vi "Switch Columns between Test tables.vi"(7 "New Table":string, 8 "error in (no error)":errorcluster, 9 "Old Column":string, 10 "Old Table":string, 11 "LV-Data.PGSQL in":refnum<class "LV-Data.PGSQL.lvclass">) -> (0 "error out":errorcluster, 2 "Result":string[][](array[string]), 3 "LV-Data.PGSQL out":refnum<class "LV-Data.PGSQL.lvclass">)   [LabVIEW 2016]
uses:
  LV-Data/src/LV-Data.PG/LV-Data.PGSQL.lvclass
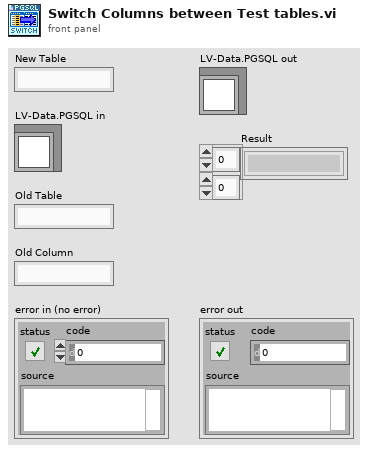
[diagram p1: front panel]
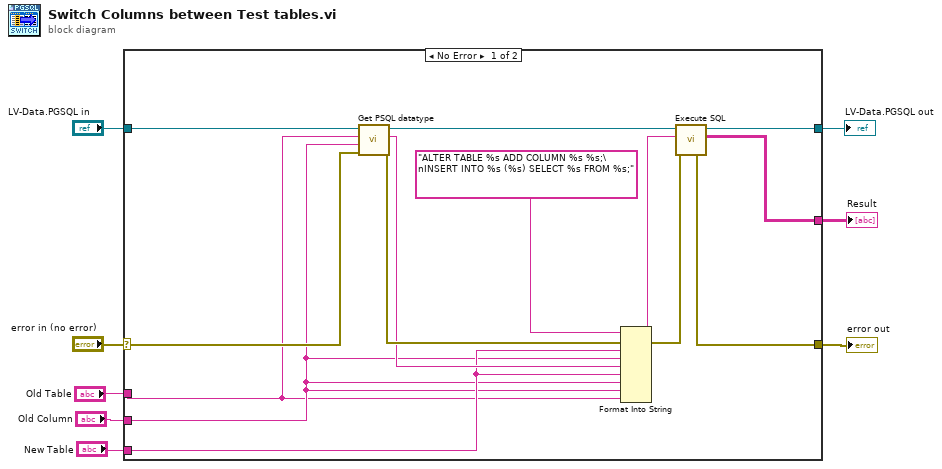
[diagram p0: block diagram]
diagram:
  n1 = case shown="No Error" "error in (no error)" {
    selector: "error in (no error)" -> [w16 w23]
    tunnel: "New Table" -> [w11 _]
    tunnel: "Old Column" -> [w10 _]
    tunnel: "LV-Data.PGSQL in" -> [w15 w24]
    tunnel: [w21 w23] -> w7
    tunnel: [w22 w24] -> w3
    tunnel: "Old Table" -> [w9 _]
    tunnel: [w19 _] -> w8
    frame No Error {
      n2 = call "Get PSQL datatype.vi"("error in (no error)"=w16, "Column"=w10, "Table"=w9, "LV-Data.PGSQL in"=w15) -> ("error out"=w13:errorcluster, "Get:Get String"=w12:string, "LV-Data.PGSQL out"=w14:refnum<class "LV-Data.PGSQL.lvclass">)  [unwired: 5 in]
      n3 = Format Into String(format string="ALTER TABLE %s ADD COLUMN %s %s;\nINSERT INTO %s (%s) SELECT %s FROM %s;", error in=w13, w11, w10, w12, w11, w10, w10, w9) -> (resulting string=w18:string, error out=w17:errorcluster)  [unwired: 1 in]
      n4 = call "Execute SQL.vi"("error in"=w17, "SQL"=w18, "Data.PG"=w14) -> ("error out"=w21:errorcluster, "Result"=w19:string[][], "Data.PG out"=w22:refnum<class "LV-Data.PGSQL.lvclass">)  [unwired: 6 in]
    }
    frame Error {
    }
  }
  "Result" <- w8
  "error out" <- w7
  "LV-Data.PGSQL out" <- w3
